vi "Measurement.WavelengthSweeping.SetConfiguration.vi"(8 "error in (no error)":errorcluster, 10 "Configuration":T1, 11 "Measurement.WavelengthSweeping":refnum<class "Measurement.WavelengthSweeping.lvclass">) -> (0 "error out":errorcluster, 3 "Measurement.WavelengthSweeping out":refnum<class "Measurement.WavelengthSweeping.lvclass">)   [LabVIEW 2017, in "Measurement.WavelengthSweeping.lvclass"]
doc: "---------------------------------------------------------------\nJKI State Machine Objects™\nhttp://jki.net/state-machine-objects/\nCopyright (C) 2005-2015, JKI <info@jki.net>\nALL RIGHTS RESERVEDJKI State Machine Objects (SMO) 1.0.0.5\nJKI - JKI\nCopyright (c) 2016, JKI"
uses:
  Measurement.WavelengthSweeping.lvclass
  Typedefs/Configuration--Cluster.ctl
  Measurement/Typedefs/Measurement.Type--Enum.ctl
  Typedefs/Configuration.Hardware--Cluster.ctl
  Measurement/Typedefs/Configuration.SMU--Cluster.ctl
  SMU/Typedefs/Configuration--Cluster.ctl
  Measurement/Typedefs/Configuration.LIA--Cluster.ctl
  LIA/Typedefs/Configuration--Cluster.ctl
  Measurement/Typedefs/Configuration.OPM--Cluster.ctl
  OPM/Typedefs/Configuration--Cluster.ctl
  Measurement/Typedefs/Configuration.OPA--Cluster.ctl
  OPA/Typedefs/Configuration--Cluster.ctl
  Measurement/Typedefs/Configuration.MC--Cluster.ctl
  MC/Typedefs/Configuration--Cluster.ctl
  Typedefs/Configuration.Measurement--Cluster.ctl
  Measurement.WavelengthSweeping.lvclass/Measurement.WavelengthSweeping.ctl
  Measurement/Measurement.lvclass
  SMU/SMU.lvclass
  LIA/LIA.lvclass
  OPM/OPM.lvclass
  OPA/OPA.lvclass
  MC/MC.lvclass
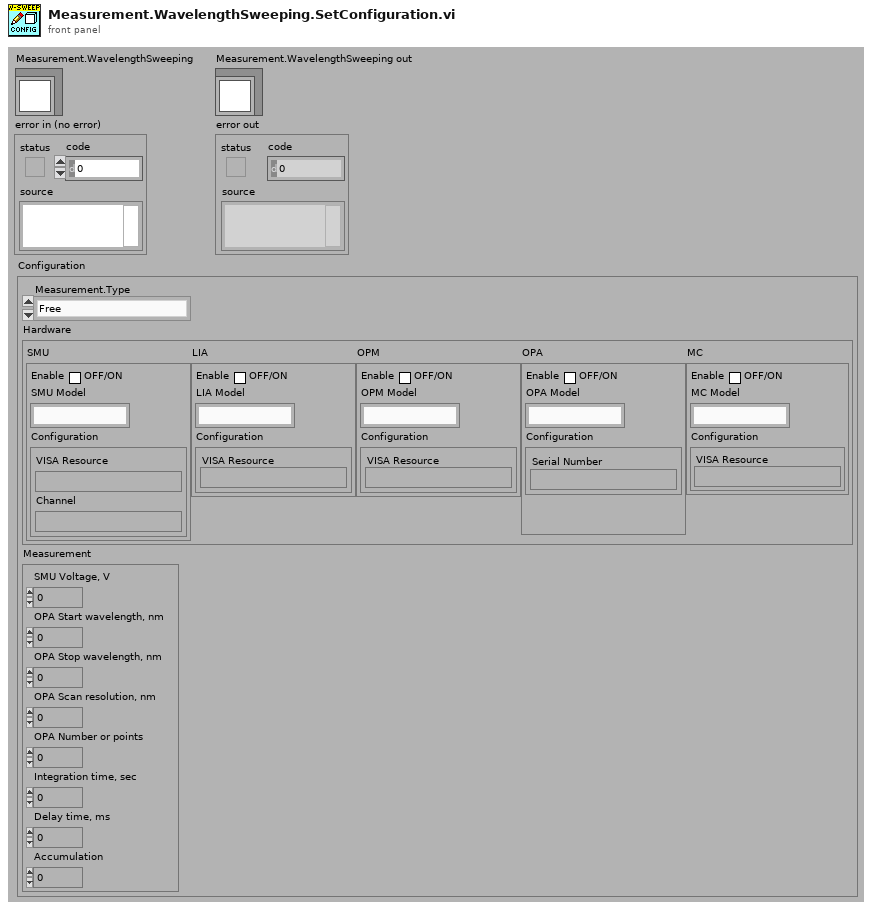
[diagram p1: front panel]
types:
  T1 = typedef "Measurement.WavelengthSweeping.lvclass/Configuration--Cluster.ctl" = cluster{"Measurement.Type":T2, "Hardware":T3, "Measurement":T14}
  T2 = typedef "Measurement.lvclass/Measurement.Type--Enum.ctl" = enum16{"Free", "I/V Curve", "Wavelength sweeping", "Photocurrent mapping"}
  T3 = typedef "Measurement.WavelengthSweeping.lvclass/Configuration.Hardware--Cluster.ctl" = cluster{"SMU":T4, "LIA":T6, "OPM":T8, "OPA":T10, "MC":T12}
  T4 = typedef "Measurement.lvclass/Configuration.SMU--Cluster.ctl" = cluster{"Enable":bool, "SMU Model":string, "Configuration":T5}
  T5 = typedef "SMU.lvclass/Configuration--Cluster.ctl" = cluster{"VISA Resource":string, "Channel":string}
  T6 = typedef "Measurement.lvclass/Configuration.LIA--Cluster.ctl" = cluster{"Enable":bool, "LIA Model":string, "Configuration":T7}
  T7 = typedef "LIA.lvclass/Configuration--Cluster.ctl" = cluster{"VISA Resource":string}
  T8 = typedef "Measurement.lvclass/Configuration.OPM--Cluster.ctl" = cluster{"Enable":bool, "OPM Model":string, "Configuration":T9}
  T9 = typedef "OPM.lvclass/Configuration--Cluster.ctl" = cluster{"VISA Resource":string}
  T10 = typedef "Measurement.lvclass/Configuration.OPA--Cluster.ctl" = cluster{"Enable":bool, "OPA Model":string, "Configuration":T11}
  T11 = typedef "OPA.lvclass/Configuration--Cluster.ctl" = cluster{"Serial Number":string}
  T12 = typedef "Measurement.lvclass/Configuration.MC--Cluster.ctl" = cluster{"Enable":bool, "MC Model":string, "Configuration":T13}
  T13 = typedef "MC.lvclass/Configuration--Cluster.ctl" = cluster{"VISA Resource":string}
  T14 = typedef "Measurement.WavelengthSweeping.lvclass/Configuration.Measurement--Cluster.ctl" = cluster{"SMU Voltage, V":dbl, "OPA Start wavelength, nm":dbl, "OPA Stop wavelength, nm":dbl, "OPA Scan resolution, nm":dbl, "OPA Number or points":u16, "Integration time, sec":dbl, "Delay time, ms":u16, "Accumulation":u16}
  T15 = typedef "Measurement.WavelengthSweeping.lvclass/PrivateData--Ref.ctl" = refnum<data-value>
  T16 = typedef "Measurement.WavelengthSweeping.lvclass/PrivateData--Cluster.ctl" = cluster{"Configuration":T1, "Dependencies":T17}
  T17 = typedef "Measurement.WavelengthSweeping.lvclass/Dependencies--Cluster.ctl" = cluster{"SMU":refnum<class "SMU.lvclass">, "LIA":refnum<class "LIA.lvclass">, "OPM":refnum<class "OPM.lvclass">, "OPA":refnum<class "OPA.lvclass">, "MC":refnum<class "MC.lvclass">}
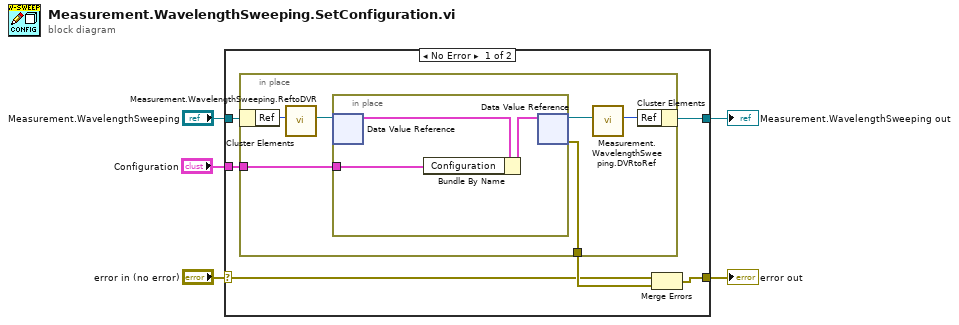
[diagram p0: block diagram]
diagram:
  n1 = case shown="No Error" "error in (no error)" {
    selector: "error in (no error)" -> [w6 w21]
    tunnel: "Measurement.WavelengthSweeping" -> [w7 w22]
    tunnel: [w8 w21] -> w4
    tunnel: [w11 w22] -> w3
    tunnel: "Configuration" -> [w10 _]
    frame No Error {
      n2 = in-place {
        in-place-border: w10 -> [w17]
        in-place-border: [w16] -> w9
        n3 = in-place-cluster #1(w7) -> ("Ref"=w15:u32)
        n4 = call "Measurement.WavelengthSweeping.ReftoDVR.vi"("Ref"=w15) -> ("Ref"=w14:T15)  [unwired: 10 in]
        n5 = in-place {
          in-place-border: w17 -> [w18]
          n6 = in-place-dvr #2(w14) -> (w20:T16)  [unwired: 1 out]
          n7 = Bundle By Name(cluster=w20, "Configuration"=w18) -> (w19:T16)
          n8 = in-place-dvr #2(w19) -> (w13:T15, w16:errorcluster)
        }
        n9 = call "Measurement.WavelengthSweeping.DVRtoRef.vi"("Ref"=w13) -> ("Ref"=w12:u32)  [unwired: 10 in]
        n10 = in-place-cluster #1("Ref"=w12) -> (w11:refnum<class "Measurement.WavelengthSweeping.lvclass">)
      }
      n11 = Merge Errors(w6, w9) -> (w8:errorcluster)
    }
    frame Error {
    }
  }
  "error out" <- w4
  "Measurement.WavelengthSweeping out" <- w3
